vi "ma_Estimate N.vi"(4 "nominal ripple":dbl=0.036315075773213946 format="%0.3e", 5 "sampling freq":dbl=1.0 format="%0.4f", 6 "Band Parameters In":T1(array[cluster])=[{"amplitude"=0.0, "lower freq"=0.0, "higher freq"=0.13333333333333333, "ripple weight"=1.0}, {"amplitude"=1.001, "lower freq"=0.16666666666666666, "higher freq"=0.3, "ripple weight"=1.0}, {"amplitude"=0.0, "lower freq"=0.3333333333333333, "higher freq"=0.5, "ripple weight"=1.0}] {"amplitude" format="%0.4f"; "lower freq" format="%0.4f"; "higher freq" format="%0.4f"; "ripple weight" format="%0.4f"}) -> (1 "all orders":dbl[](array[numeric]) format="%0.2f", 2 "order":i32 min=0)   [LabVIEW 2020, in "NI_MAPro.lvlib"]
uses:
  NI_MAPro.lvlib
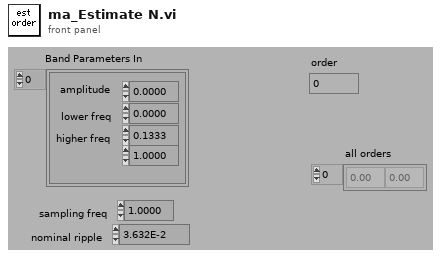
[diagram p1: front panel]
types:
  T1 = cluster{"amplitude":dbl, "lower freq":dbl, "higher freq":dbl, "ripple weight":dbl}[]
  T2 = cluster{"amplitude":dbl, "lower freq":dbl, "higher freq":dbl, "ripple weight":dbl}
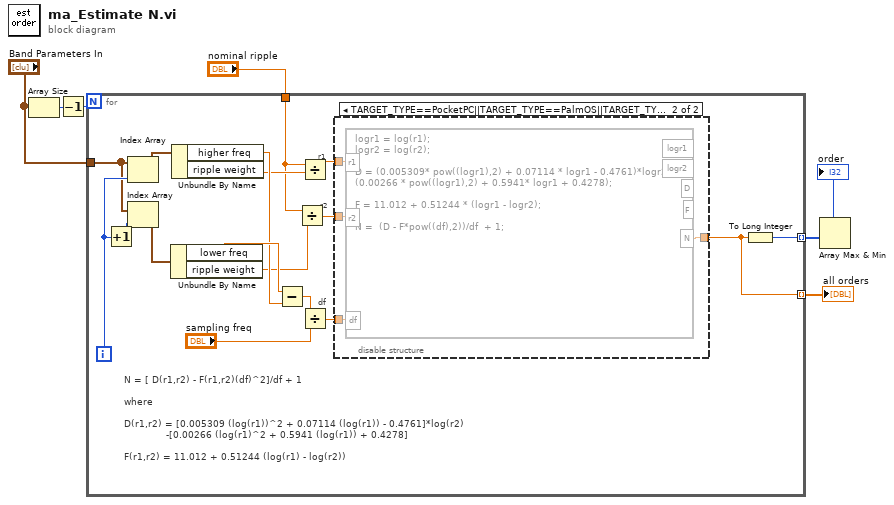
[diagram p0: block diagram]
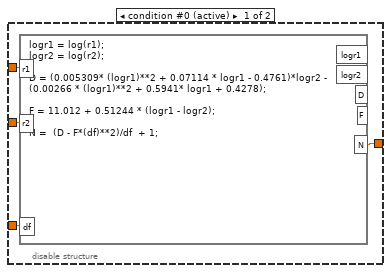
[diagram p2: hidden frame]
diagram:
  n1 = Array Size(array="Band Parameters In") -> (size(s)=w7:i32)
  n2 = Decrement(x=w7) -> (x-1=w6:i32)
  n3 = for {
    N: w6 -> [_]
    tunnel: "Band Parameters In" -> [w22]
    tunnel: [w9] -> w1 mode=indexing
    tunnel: "nominal ripple" -> [w13]
    tunnel: [w8] -> w2 mode=indexing
    i -> [w24]
    # "r2"
    # "r1"
    # "N = [ D(r1,r2) - F(r1,r2)(df)^2]/df + 1\n\nwhere\n\nD(r1,r2) = [0.005309 (log(r1))^2 + 0.07114 (log(r1)) - 0.4761]*log(r2)\n              -[0.00266 (log(r1)^2 + 0.5941 (log(r1)) + 0.4278]\n\nF(r1,r2) = 11.012 + 0.51244 (log(r1) - log(r2))"
    # "df"
    n4 = Increment(x=w24) -> (x+1=w23:i32)
    n5 = Index Array(array=w22, index=w24) -> (element=w21:T2)
    n6 = Index Array(array=w22, index=w23) -> (element=w20:T2)
    n7 = Unbundle By Name(w20) -> ("lower freq"=w19:dbl, "ripple weight"=w14:dbl)
    n8 = Unbundle By Name(w21) -> ("higher freq"=w18:dbl, "ripple weight"=w15:dbl)
    n9 = Subtract(x=w19, y=w18) -> (x-y=w17:dbl)
    n10 = Divide(x=w13, y=w14) -> (x/y=w11:dbl)
    n11 = Divide(x=w13, y=w15) -> (x/y=w12:dbl)
    n12 = Divide(x=w17, y="sampling freq") -> (x/y=w10:dbl)
    n13 = disable-structure shown="TARGET_TYPE==PocketPC||TARGET_TYPE==PalmOS||TARGET_TYPE==Embedded" {
      disable-tunnel: w12 -> [w28 w32]
      disable-tunnel: w11 -> [w27 w31]
      disable-tunnel: w10 -> [w26 w30]
      disable-tunnel: [w25 w29] -> w8
      frame condition #0 (active) {
        n14 = formula code="logr1 = log(r1);\nlogr2 = log(r2);\n\nD = (0.005309* (logr1)**2 + 0.07114 * logr1 - 0.4761)*logr2 - (0.00266 * (logr1)**2 + 0.5941* logr1 + 0.4278);\n\nF = 11.012 + 0.51244 * (logr1 - logr2);\n\nN =  (D - F*(df)**2)/df  + 1;"("r1"=w28, "r2"=w27, "df"=w26) -> ("N"=w25:dbl)  [unwired: 4 out]
      }
      frame condition #1 {
        n15 = formula code="logr1 = log(r1);\nlogr2 = log(r2);\n\nD = (0.005309* pow((logr1),2) + 0.07114 * logr1 - 0.4761)*logr2 - (0.00266 * pow((logr1),2) + 0.5941* logr1 + 0.4278);\n\nF = 11.012 + 0.51244 * (logr1 - logr2);\n\nN =  (D - F*pow((df),2))/df  + 1;"("r1"=w32, "r2"=w31, "df"=w30) -> ("N"=w29:dbl)  [unwired: 4 out]
      }
    }
    n16 = To Long Integer(number=w8) -> (32bit integer=w9:i32)
  }
  "all orders" <- w2
  n17 = Array Max & Min(array=w1) -> (max value=→"order":i32)  [unwired: 3 out]
